vi "To and From Array Test.vi"() -> (0 "error out":errorcluster, 2 "Lines Equal":bool, 3 "Class Equal":bool)   [LabVIEW 2015, in "PID Module 2 tests.lvlib"]
uses:
  PID Module 2 tests.lvlib
  module/configuration/PID Module 2 configuration.lvclass/PID Module 2 configuration.ctl
  <vilib>/NI/Tag Bus/tag/tag descriptor.lvclass/tag descriptor.ctl
  <vilib>/NI/Tag Bus/tag/default value polymorphs/read default value Double.vi
  <vilib>/NI/Tag Bus Module Framework/channel/TBM channel.lvclass
  module/configuration/PID Module 2 configuration.lvclass
  <vilib>/NI/Tag Bus/tag/tag descriptor.lvclass
panel:
  out "Array 4":string[](array[string])
  out "Array 3":string[](array[string])
  out "x = y?":T1(array[cluster])
  out "Array 2":string[][](array[string])
  out "Array":string[][](array[string])
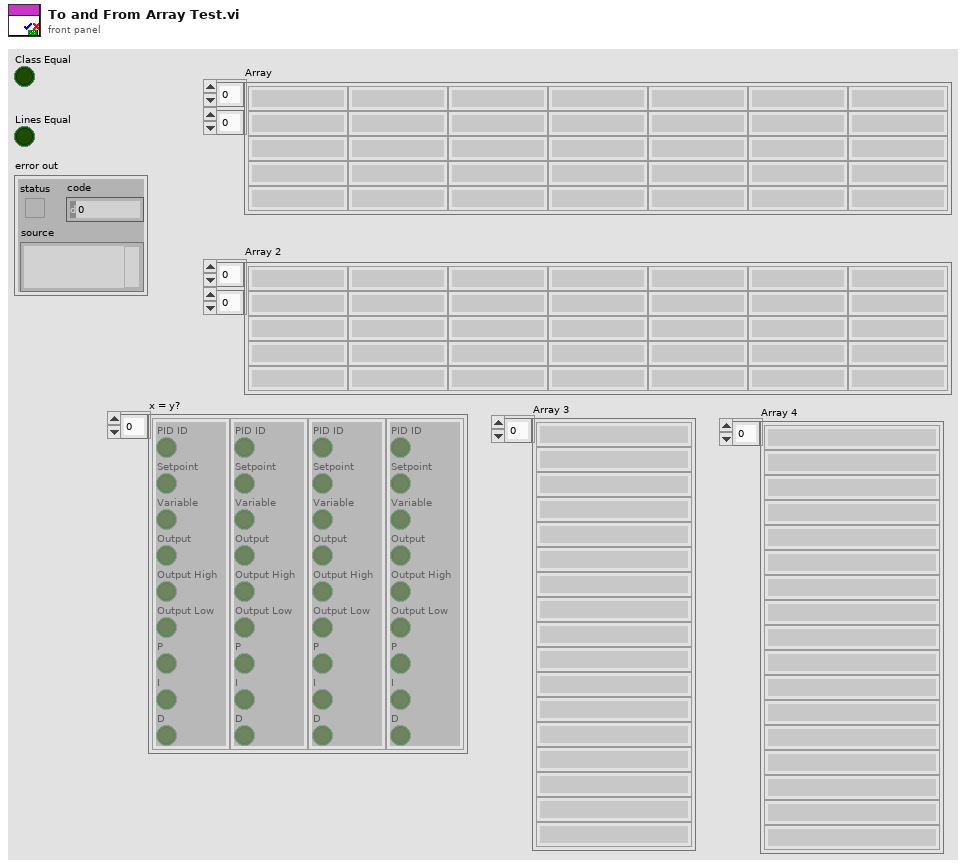
[diagram p1: front panel]
types:
  T1 = cluster{"PID ID":bool, "Setpoint":bool, "Variable":bool, "Output":bool, "Output High":bool, "Output Low":bool, "P":bool, "I":bool, "D":bool}[]
  T2 = typedef "PID Module 2 configuration.lvclass/Line.ctl" = cluster{"PID ID":string, "Setpoint":refnum<class "TBM channel.lvclass">, "Variable":refnum<class "TBM channel.lvclass">, "Output":refnum<class "TBM channel.lvclass">, "Output High":refnum<class "TBM channel.lvclass">, "Output Low":refnum<class "TBM channel.lvclass">, "P":refnum<class "TBM channel.lvclass">, "I":refnum<class "TBM channel.lvclass">, "D":refnum<class "TBM channel.lvclass">}
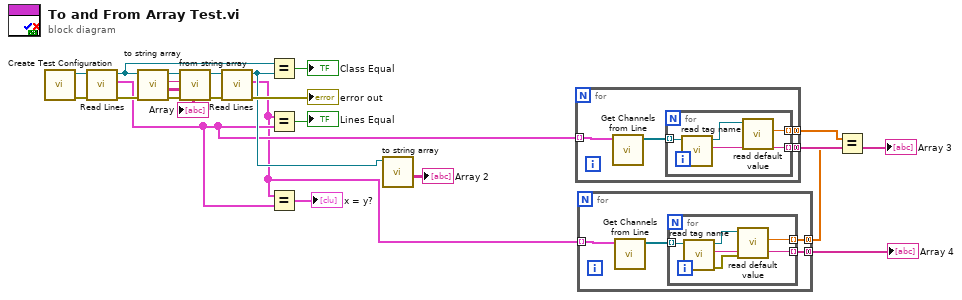
[diagram p0: block diagram]
diagram:
  n1 = call "Create Test Configuration.vi"() -> ("error out"=w14:errorcluster, "Module Configuration"=w15:refnum<class "PID Module 2 configuration.lvclass">)  [unwired: 6 in, 4 out]
  n2 = call "Read Lines.vi"("error in (no error)"=w14, "PID Module 2 configuration in"=w15) -> ("error out"=w16:errorcluster, "Lines"=w7:T2[], "PID Module 2 configuration out"=w13:refnum<class "PID Module 2 configuration.lvclass">)  [unwired: 7 in]
  n3 = call-dynamic "to string array.vi"("error in (no error)"=w16, "PID Module 2 configuration in"=w13) -> ("error out"=w22:errorcluster, "Array"=w21:string[][], "version"=w20:string, "PID Module 2 configuration out"=w19:refnum<class "PID Module 2 configuration.lvclass">)  [unwired: 6 in]
  "Array" <- w21
  n4 = call-dynamic "from string array.vi"("error in (no error)"=w22, "String Array"=w21, "version"=w20, "PID Module 2 configuration in"=w19) -> ("error out"=w17:errorcluster, "PID Module 2 configuration out"=w18:refnum<class "PID Module 2 configuration.lvclass">)  [unwired: 6 in]
  n5 = call "Read Lines.vi"("error in (no error)"=w17, "PID Module 2 configuration in"=w18) -> ("error out"=→"error out":errorcluster, "Lines"=w3:T2[], "PID Module 2 configuration out"=w9:refnum<class "PID Module 2 configuration.lvclass">)  [unwired: 7 in]
  n6 = Equal?(x=w13, y=w9) -> (x = y?=→"Class Equal":bool)
  n7 = Equal?(x=w3, y=w7) -> (x = y?=→"Lines Equal":bool)
  n8 = Equal?(x=w3, y=w7) -> (x = y?=→"x = y?":T1)
  n9 = call-dynamic "to string array.vi"("PID Module 2 configuration in"=w9) -> ("Array"=→"Array 2":string[][])  [unwired: 7 in, 3 out]
  n10 = for {
    tunnel: w7 -> [w26] mode=indexing
    tunnel: [w24] -> w5 mode=concatenating
    tunnel: [w23] -> w2 mode=concatenating
    n11 = call "Get Channels from Line.vi"("Line"=w26) -> ("Channels"=w25:refnum<class "TBM channel.lvclass">[])  [unwired: 10 in]
    n12 = for {
      tunnel: w25 -> [w30] mode=indexing
      tunnel: [w29] -> w24 mode=indexing
      tunnel: [w27] -> w23 mode=indexing
      n13 = call <vilib>:"read tag name.vi"("system tag in"=w30) -> ("name"=w29:string, "system tag out"=w28:refnum<class "TBM channel.lvclass">)  [unwired: 8 in, 1 out]
      n14 = call-poly <vilib>:"read default value.vi"("system tag in"=w28) -> ("default value"=w27:dbl)  [unwired: 7 in, 3 out]
    }
  }
  "Array 3" <- w5
  n15 = for {
    tunnel: w3 -> [w34] mode=indexing
    tunnel: [w32] -> w4 mode=concatenating
    tunnel: [w31] -> w1 mode=concatenating
    n16 = call "Get Channels from Line.vi"("Line"=w34) -> ("Channels"=w33:refnum<class "TBM channel.lvclass">[])  [unwired: 10 in]
    n17 = for {
      tunnel: w33 -> [w39] mode=indexing
      tunnel: [w38] -> w32 mode=indexing
      tunnel: [w35] -> w31 mode=indexing
      n18 = call <vilib>:"read tag name.vi"("system tag in"=w39) -> ("error out"=w37:errorcluster, "name"=w38:string, "system tag out"=w36:refnum<class "TBM channel.lvclass">)  [unwired: 8 in]
      n19 = call-poly <vilib>:"read default value.vi"("error in"=w37, "system tag in"=w36) -> ("default value"=w35:dbl)  [unwired: 6 in, 3 out]
    }
  }
  "Array 4" <- w4
  n20 = Equal?(x=w2, y=w1) -> ()  [unwired: 1 out]
